vi "joyref (SubVI).vi"(1 "ZETA":dbl[](array[numeric])=[1.0, 1.0, 1.0, 1.0], 2 "dt":dbl=0.2, 3 "OMEGA":dbl[](array[numeric])=[0.5, 0.5, 0.5, 0.5], 4 "R":dbl[](array[numeric])=[0.0, 0.0, 0.0, 0.0], 5 "Max acc":dbl[](array[numeric])=[1.0, 1.0, 1.0, 1.0], 6 "Max vel":dbl[](array[numeric])=[2.0, 2.0, 2.0, 2.0]) -> (0 "Eta des":dbl[](array[numeric]))   [LabVIEW 2010]
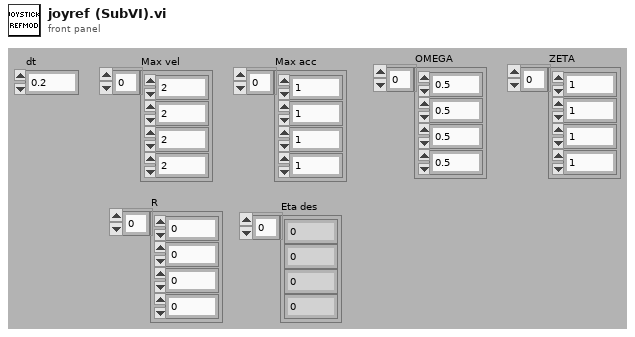
[diagram p1: front panel]
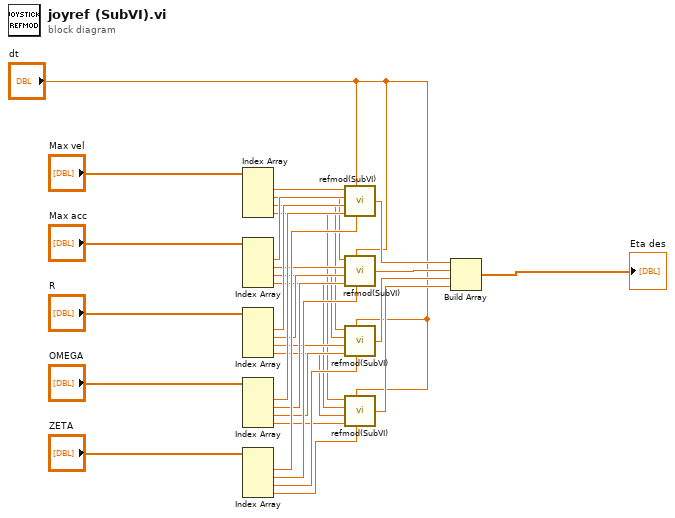
[diagram p0: block diagram]
diagram:
  n1 = Index Array(array="Max vel") -> (element #1=w7:dbl, element #2=w8:dbl, element #3=w9:dbl, element #4=w10:dbl)  [unwired: 4 in]
  n2 = Index Array(array="Max acc") -> (element #1=w11:dbl, element #2=w12:dbl, element #3=w13:dbl, element #4=w14:dbl)  [unwired: 4 in]
  n3 = Index Array(array="R") -> (element #1=w15:dbl, element #2=w16:dbl, element #3=w17:dbl, element #4=w18:dbl)  [unwired: 4 in]
  n4 = Index Array(array="OMEGA") -> (element #1=w19:dbl, element #2=w20:dbl, element #3=w21:dbl, element #4=w22:dbl)  [unwired: 4 in]
  n5 = Index Array(array="ZETA") -> (element #1=w23:dbl, element #2=w24:dbl, element #3=w25:dbl, element #4=w26:dbl)  [unwired: 4 in]
  n6 = call "refmod(SubVI).vi"("zeta"=w23, "dt"="dt", "omega"=w19, "r"=w15, "max acc"=w11, "max vel"=w7) -> ("output"=w27:dbl)
  n7 = call "refmod(SubVI).vi"("zeta"=w24, "dt"="dt", "omega"=w20, "r"=w16, "max acc"=w12, "max vel"=w8) -> ("output"=w28:dbl)
  n8 = call "refmod(SubVI).vi"("zeta"=w25, "dt"="dt", "omega"=w21, "r"=w17, "max acc"=w13, "max vel"=w9) -> ("output"=w29:dbl)
  n9 = call "refmod(SubVI).vi"("zeta"=w26, "dt"="dt", "omega"=w22, "r"=w18, "max acc"=w14, "max vel"=w10) -> ("output"=w30:dbl)
  n10 = Build Array(w27, w28, w29, w30) -> (→"Eta des":dbl[])
